vi "PCAN_INIT.vi"(8 "error in (no error)":errorcluster, 10 "Msg Type":i32(ring) items=["standart", "extended"], 11 "BTR0BTR1":u16(ring)=20 items=["1M"=20, "500K"=28, "250K"=284, "125K"=796, "100K"=17199, "50K"=18223, "20K"=21295, "10K"=26415, "5K"=32639]) -> (0 "error out":errorcluster, 3 "error":T1 items=["CAN_ERR_OK"=0, "CAN_ERR_XMTFULL"=1, "CAN_ERR_OVERRUN"=2, "CAN_ERR_BUSLIGHT"=4, "CAN_ERR_BUSHEAVY"=8, "CAN_ERR_BUSOFF"=16, "CAN_ERR_QRCVEMPTY"=32, "CAN_ERR_QOVERRUN"=64, "CAN_ERR_QXMTFULL"=128, "CAN_ERR_REGTEST"=256, "CAN_ERR_NOVXD"=512, "CAN_ERR_RESOURCE"=8192, "CAN_ERR_ILLPARAMTYPE"=16384, "CAN_ERR_ILLPARAMVAL"=32768])   [LabVIEW 2016]
doc: "///////////////////////////////////////////////////////////////////////////////\n// CAN_Init()\n// Aktiviert eine Hardware, macht Registertest des 82C200/SJA1000,\n// teilt einen Sendepuffer und ein HardwareHandle zu.\n// Programmiert Konfiguration der Sende/Empfangstreiber.\n// Controller bleibt im Resetzustand.\n// Uebergibt die Baudratenregister\n// Wenn CANMsgType=0 ---> 11Bit ID Betrieb\n// Wenn CANMsgType=1 ---> 11/29Bit ID Betrieb\n// moegliche Fehler: NOVXD ILLHW REGTEST RESOURCE\n// \n\nDWORD __stdcall CAN_Init(WORD wBTR0BTR1, int CANMsgType); // Baudrate"
uses:
  PCAN_ERROR.ctl
  PCAN_USB.DLL
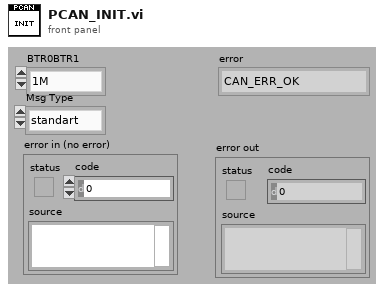
[diagram p1: front panel]
types:
  T1 = typedef "PCAN_ERROR.ctl" = i32
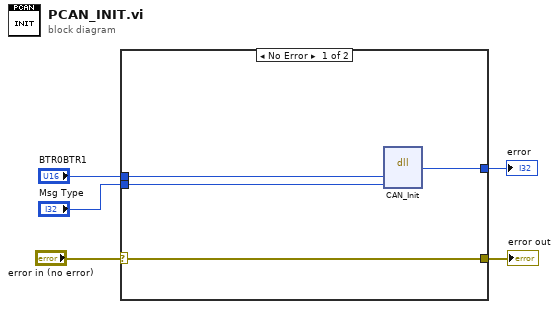
[diagram p0: block diagram]
diagram:
  n1 = case shown="No Error" "error in (no error)" {
    selector: "error in (no error)" -> [w6 w10]
    tunnel: "BTR0BTR1" -> [w9 _]
    tunnel: "Msg Type" -> [w8 _]
    tunnel: [w7 _] -> w3
    tunnel: [w6 w10] -> w1
    frame No Error {
      n2 = dll-call lib="D:/LabView/08_PCAN&Measurement/PCAN_Driver/PCAN_USB.DLL" fn="CAN_Init"("wBTR0BTR1"=w9, "CANMsgType"=w8) -> ("return type"=w7:i32)  [unwired: 5 in, 2 out]
    }
    frame Error {
    }
  }
  "error" <- w3
  "error out" <- w1
